vi "Acquire Status of Dependency Targets.vi"(8 "Error In":errorcluster) -> (0 "Error Out":errorcluster, 1 "Success?":bool)   [LabVIEW 2019, in "Project.Dependencies Finder.lvlib"]
doc: "Remove all local Dependency Finder files and folders (deleting [AppData]\\HDH\\Dependency Finder)\n\n2020-12-21: Henrik Dueholm Hansen"
uses:
  Project.Dependencies Finder.lvlib
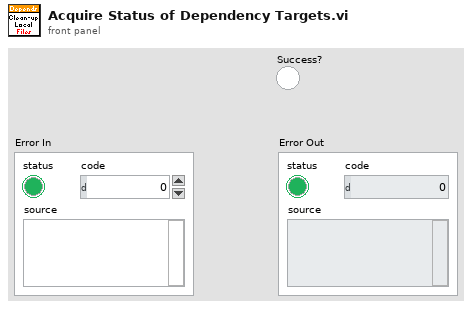
[diagram p1: front panel]
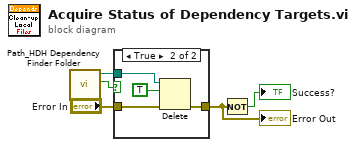
[diagram p0: block diagram]
diagram:
  n1 = call "Path_HDH Dependency Finder Folder.vi"() -> ("Success?"=w5:bool, "HDH\\VIPM path"=w4:path)  [unwired: 10 in]
  n2 = case shown="True" w5 {
    tunnel: w4 -> [_ w10]
    tunnel: "Error In" -> [w6 w8]
    tunnel: [w6 w7] -> w2
    frame False {
    }
    frame True {
      n3 = Delete(path (use dialog)=w10, entire hierarchy (F)=TRUE, error in=w8) -> (error out=w7:errorcluster)  [unwired: 2 in, 2 out]
    }
  }
  "Error Out" <- w2
  n4 = Not(x=w2) -> (.not. x?=→"Success?":bool)
